vi "find_midpoint_retroreflective.vi"(3 "Cluster":T1, 4 "reset_tape":bool, 5 "run_time":fxp<+,40,40>) -> (0 "timeOfMidpoint":fxp<+,41,40>, 1 "tape_count":u8, 2 "complete":bool)   [LabVIEW 2018]
uses:
  comp-src/validated_bool.ctl
  <vilib>/rvi/FXPMathLib/FxpAdd/XNode/nifxpmath_Add.xnode
  <vilib>/rvi/FXPMathLib/FxpMul/XNode/nifxpmath_Multiplier.xnode
  <vilib>/rvi/FXPMathLib/sim/FxpSim.dll
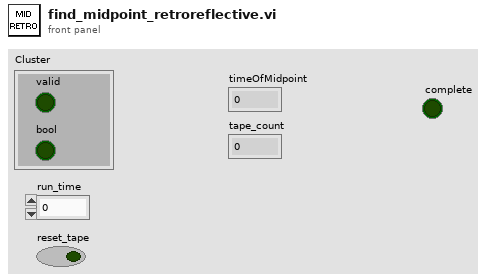
[diagram p1: front panel]
types:
  T1 = typedef "validated_bool.ctl" = cluster{"valid":bool, "bool":bool}
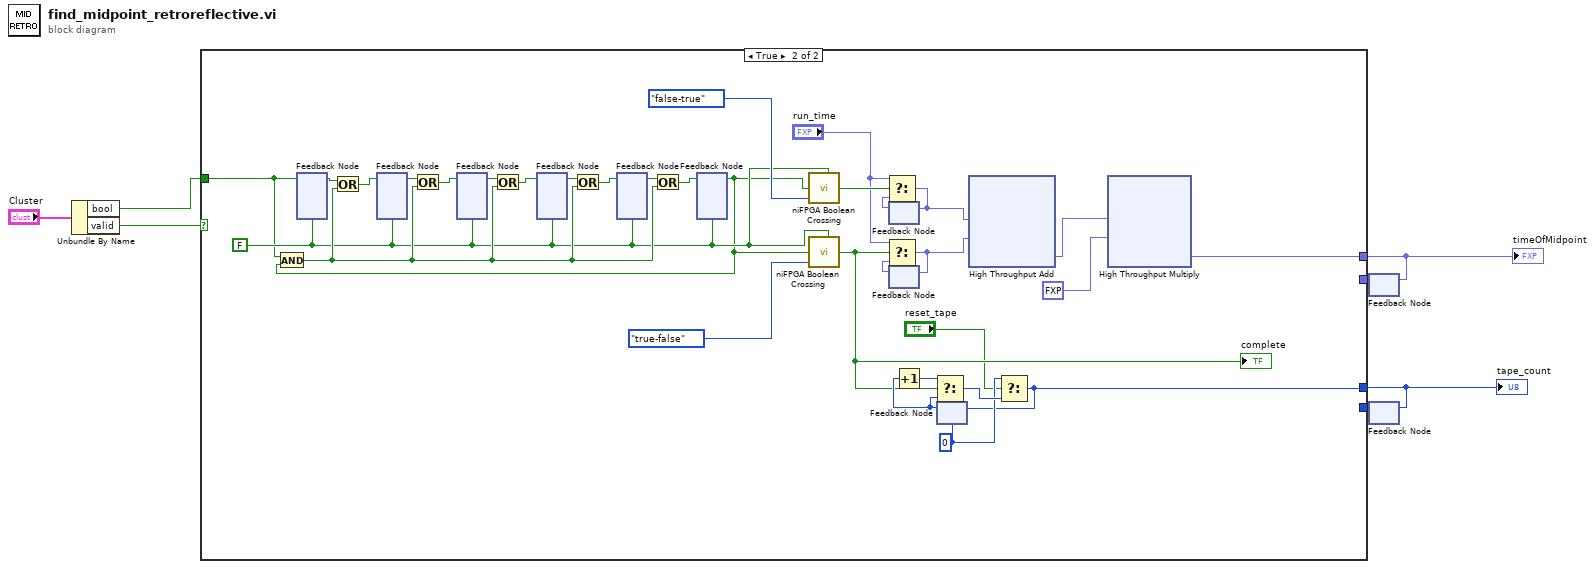
[diagram p0: block diagram]
diagram:
  n1 = Unbundle By Name("Cluster") -> ("bool"=w7:bool, "valid"=w6:bool)
  n2 = feedback #1() -> (w1:fxp<+,41,40>)  [unwired: 1 in]
  n3 = feedback #2() -> (w2:u8)  [unwired: 1 in]
  n4 = case shown="True" w6 {
    tunnel: w7 -> [_ w18]
    tunnel: [w9 w11] -> w3
    tunnel: [w8 w10] -> w4
    tunnel: w2 -> [w9 _]
    tunnel: w1 -> [w8 _]
    frame False {
    }
    frame True {
      w13 = u8 0
      w29 = FALSE
      n5 = feedback #3(w29) -> (w41:bool)
      n6 = feedback-in #3(w18) -> ()
      n7 = feedback #4(w29) -> (w40:bool)
      n8 = feedback #5(w29) -> (w39:bool)
      n9 = feedback #6(w29) -> (w38:bool)
      n10 = feedback #7(w29) -> (w34:bool)
      n11 = feedback #8(w29) -> (w28:bool)
      n12 = And(x=w18, y=w28) -> (x .and. y?=w31:bool)
      n13 = Or(x=w41, y=w31) -> (x .or. y?=w35:bool)
      n14 = feedback-in #4(w35) -> ()
      n15 = Or(x=w40, y=w31) -> (x .or. y?=w36:bool)
      n16 = feedback-in #5(w36) -> ()
      n17 = Or(x=w39, y=w31) -> (x .or. y?=w37:bool)
      n18 = feedback-in #6(w37) -> ()
      n19 = Or(x=w38, y=w31) -> (x .or. y?=w33:bool)
      n20 = feedback-in #7(w33) -> ()
      n21 = Or(x=w34, y=w31) -> (x .or. y?=w32:bool)
      n22 = feedback-in #8(w32) -> ()
      n23 = call <vilib>:"niFPGA Boolean Crossing.vi"("input"=w28, "direction"=enum8{"either", "false-true", "true-false"}."false-true", "initialize"=w29) -> ("crossing"=w27:bool)  [unwired: 6 in]
      n24 = call <vilib>:"niFPGA Boolean Crossing.vi"("input"=w28, "direction"=enum8{"either", "false-true", "true-false"}."true-false", "initialize"=w29) -> ("crossing"=w14:bool)  [unwired: 6 in]
      "complete" <- w14
      n25 = feedback #9() -> (w25:fxp<+,40,40>)  [unwired: 1 in]
      n26 = Select(t="run_time", s=w27, f=w25) -> (s? t:f=w22:fxp<+,40,40>)
      n27 = feedback-in #9(w22) -> ()
      n28 = feedback #10() -> (w26:fxp<+,40,40>)  [unwired: 1 in]
      n29 = Select(t="run_time", s=w14, f=w26) -> (s? t:f=w21:fxp<+,40,40>)
      n30 = feedback-in #10(w21) -> ()
      n31 = feedback #11(w13) -> (w15:u8)
      n32 = Increment(x=w15) -> (x+1=w16:u8)
      n33 = Select(t=w16, s=w14, f=w15) -> (s? t:f=w17:u8)
      n34 = xnode ("High Throughput Add")("x"=w22, "y"=w21) -> ("x+y"=w20:fxp<+,41,41>)
      n35 = Select(t=w13, s="reset_tape", f=w17) -> (s? t:f=w11:u8)
      n36 = feedback-in #11(w11) -> ()
      n37 = xnode ("High Throughput Multiply")("x"=w20, "y"=fxp<+,1,0> 0.5) -> ("x*y"=w10:fxp<+,41,40>)
    }
  }
  "tape_count" <- w3
  "timeOfMidpoint" <- w4
  n38 = feedback-in #1(w4) -> ()
  n39 = feedback-in #2(w3) -> ()
